vi "PythonVersion.vi"() -> ()   [LabVIEW 2019]
panel:
  in  "Python version":string="3.7"
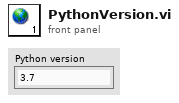
[diagram p1: front panel]
diagram:
